vi "Update DI DAQ IO Group.vi"(7 "dCVT DAQDict":T2, 8 "error in (no error)":errorcluster, 9 "DI in":bool[](array[boolean]), 10 "DI channels":T3[](array[typedef]), 11 "DIO ClusterArray":T1[](array[typedef])) -> (0 "error out":errorcluster, 3 "DIO ClusterArray out":T1[](array[typedef]), 5 "dCVT DAQDict out":T2)   [LabVIEW 2020, in "DAQDict.lvlib"]
uses:
  DAQDict.lvlib
  support/IONameNode--cluster.ctl
  <vilib>/TELLC/Dynamic CVT API/TD Dynamic CVT DVR--ref.ctl
  support/DIO ClusterArray Element--cluster.ctl
  support/BRS_DI - New.ctl
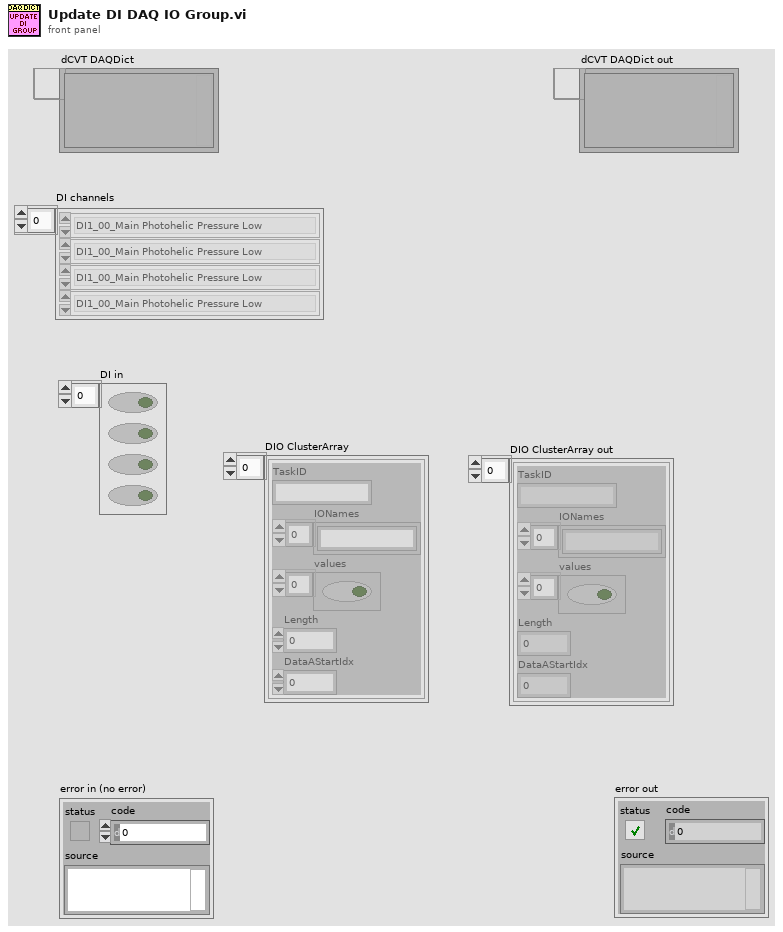
[diagram p1: front panel]
types:
  T1 = typedef "DIO ClusterArray Element--cluster.ctl" = cluster{"TaskID":string, "IONames":string[], "values":bool[], "Length":i32, "DataAStartIdx":i32}
  T2 = typedef "TD Dynamic CVT DVR--ref.ctl" = refnum<data-value>
  T3 = typedef "BRS_DI - New.ctl" = enum16{"DI1_00_Main Photohelic Pressure Low", "DI1_01_Main Photohelic Pressure High", "DI1_02_Main E-Stop Circuit OK", "DI1_03_EMO Circuit OK", "DI1_04_Nitrogen Top Valve Open", "DI1_05_Nitrogen Bottom Valve Open", "DI1_06_Nitrogen Pressure OK", "DI1_07_CDA Pressure OK", "DI1_08_Vacuum OK", "DI1_09_Aligner Home", "DI1_10_Aligner Reticle Present", "DI1_11_Main Door Interlock Solenoid Closed", "DI1_12_Main Door Closed", "DI1_13_Main Robot $ALARM_STOP", "DI1_14_Main Robot $IN_HOME", "DI1_15_Main Robot $PERI_RDY", "DI1_16_Main Robot $TCP_OPEN", "DI1_17_Main End Eff Open", "DI1_18_Main End Eff Closed", "DI1_19_Main Reticle Presence sensor-Arm-Right", "DI1_20_Spare_1", "DI1_21_Main Reticle Presence sensor-Arm-Left", "DI1_22_EXP1 XFR Reticle Present", "DI1_23_EXP2 XFR Reticle Present", "DI1_24_Main Robot $EXT (External Mode ON)", "DI1_25_Main Robot $PRO_ACT (Program Active)", "DI1_26_Main Robot $PRO_MOVE (Motion Active)", "DI1_27_Main Robot Spare1", "DI1_28_Main Robot Spare2", "DI1_29_Main Robot Spare3", "DI1_30_Spare_2", "DI1_31_Spare_3", "DI2_00_ASML_RSP LP 1 Pod Presence", "DI2_01_Spare_4", "DI2_02_ASML_RSP LP 2 Pod Presence", "DI2_03_Spare_5", "DI2_04_ASML_RSP LP 3 Pod Presence", "DI2_05_Spare_6", "DI2_06_Spare_7", "DI2_07_Manual Loadport 1 Pod Present", "DI2_08_Manual Loadport 1 Pod Capture", "DI2_09_Manual Loadport 1 Arm in Open Position", "DI2_10_Manual Loadport 1 Arm in Closed Position", "DI2_11_Manual Loadport 1 Lid Capture", "DI2_12_Manual Loadport 1 Door Closed", "DI2_13_Manual Loadport 1 Reticle Present", "DI2_14_Manual Loadport 1 Lid Present on Arm", "DI2_15_MLP Spare Input", "DI2_16_Pod Buffer Inbound Pod Present", "DI2_17_Pod Buffer Outbound Pod Present", "DI2_18_Pod Buffer Door Closed", "DI2_19_Pod Buffer Light Curtain OK", "DI2_20_Pod Buffer Light Curtain Misc Input", "DI2_21_Pod Buffer Gripper Pod Present", "DI2_22_Pod Buffer Gripper open", "DI2_23_Pod Buffer Gripper closed", "DI2_24_FFU Pressure sensor 1", "DI2_25_FFU Pressure sensor 2", "DI2_26_FFU Pressure sensor 3", "DI2_27_FFU Pressure sensor 4", "DI2_28_FFU Pressure sensor 5", "DI2_29_FFU Pressure sensor 6", "DI2_30_FFU Pressure sensor 7", "DI2_31_FFU Pressure sensor 8", "DI3_00_Exp1 Photohelic Pressure Low", "DI3_01_Exp1 Photohelic Pressure High", "DI3_02_Main E-Stop Circuit OK", "DI3_03_Spare_1", "DI3_04_Exp1 Door Interlock Solenoid Closed", "DI3_05_Exp1 Door Closed", "DI3_06_Spare_2", "DI3_07_Spare_3", "DI3_08_Spare_4", "DI3_09_Spare_5", "DI3_10_Exp1 End Eff Open", "DI3_11_Exp1 End Eff Closed", "DI3_12_Exp1 Reticle Presence sensor-Arm-Right", "DI3_13_Exp1 Robot $ALARM_STOP", "DI3_14_Exp1 Robot $IN_HOME", "DI3_15_Exp1 Robot $PERI_RDY", "DI3_16_Exp1 Robot $TCP_OPEN", "DI3_17_Exp1 Reticle Presence sensor-Arm-Left", "DI3_18_Exp1 FFU Pressure sensor 1", "DI3_19_Exp1 FFU Pressure sensor 2", "DI3_20_Exp1 FFU Pressure sensor 3", "DI3_21_Exp1 FFU Pressure sensor 4", "DI3_22_Exp1 FFU Pressure sensor 5", "DI3_23_Exp1 FFU Pressure sensor 6", "DI3_24_Exp1 Robot $EXT (External Mode ON)", "DI3_25_Exp1 Robot $PRO_ACT (Program Active)", "DI3_26_Exp1 Robot $PRO_MOVE (Motion Active)", "DI3_27_Exp1 FFU Pressure sensor 7", "DI3_28_Exp1 FFU Pressure sensor 8", "DI3_29_Exp1 output Spare 1", "DI3_30_Exp1 output Spare 2", "DI3_31_Exp1 output Spare 3"}
  T4 = typedef "IONameNode--cluster.ctl" = cluster{"IOName":string, "value":bool, "IO Type":enum16{"N/A", "DI", "DO"}, "TaskID":string, "data Idx":i32}
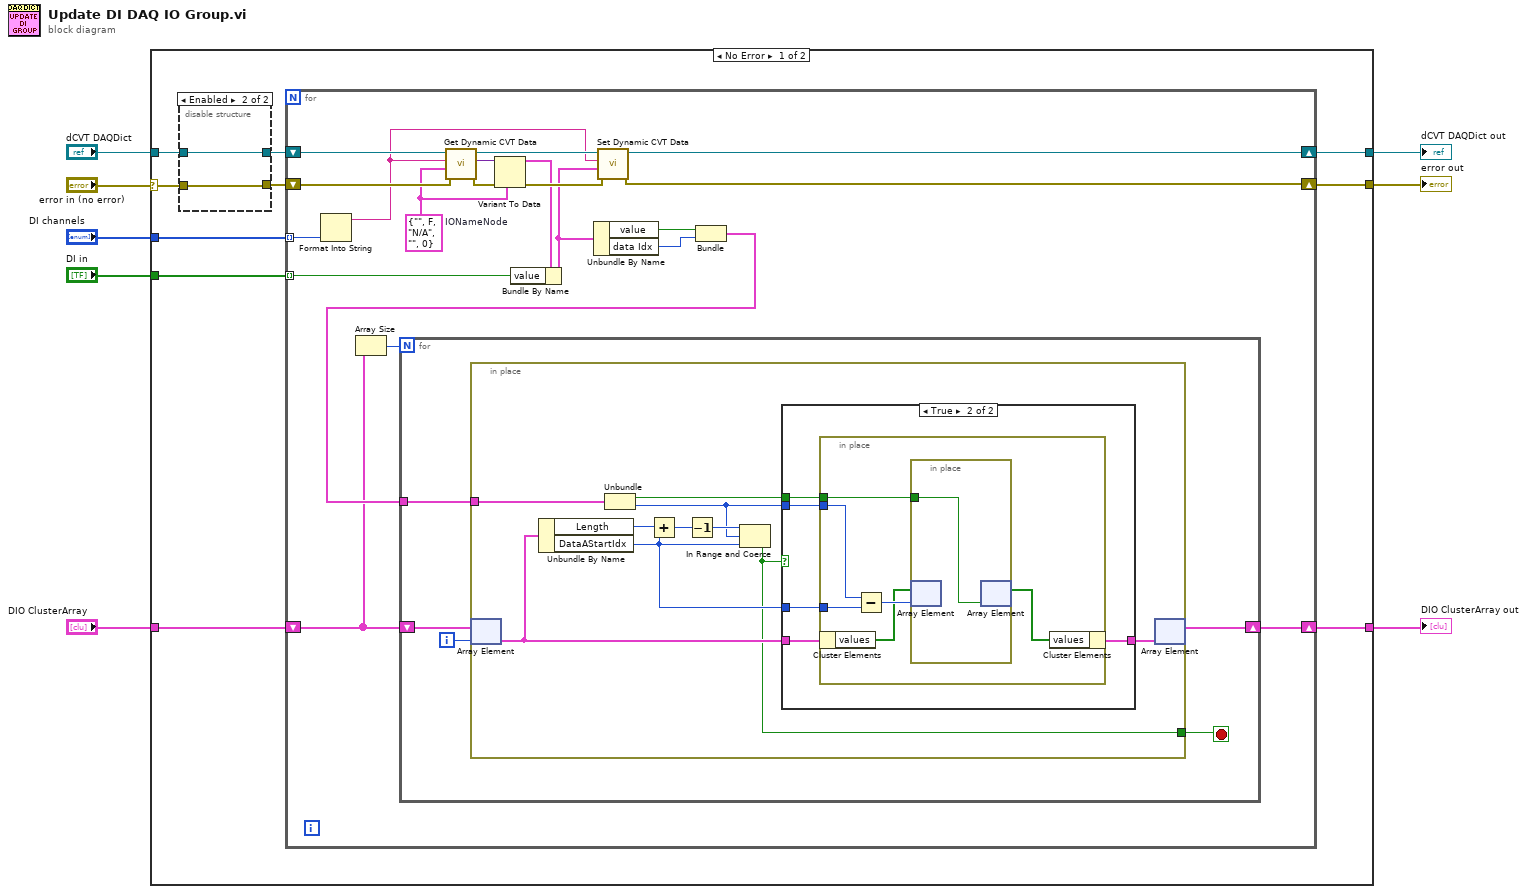
[diagram p0: block diagram]
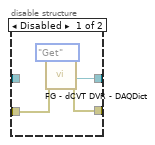
[diagram p2: hidden frame]
diagram:
  n1 = case shown="No Error" "error in (no error)" {
    selector: "error in (no error)" -> [w17 w75]
    tunnel: [w15 w75] -> w8
    tunnel: "DI channels" -> [w16 _]
    tunnel: [w14 w74] -> w5
    tunnel: "dCVT DAQDict" -> [w12 w74]
    tunnel: "DI in" -> [w11 _]
    tunnel: "DIO ClusterArray" -> [w10 w73]
    tunnel: [w9 w73] -> w1
    frame No Error {
      n2 = disable-structure shown="Enabled" {
        disable-tunnel: [w21 w23] -> w18
        disable-tunnel: w17 -> [w20 w23]
        disable-tunnel: [w19 w24] -> w13
        disable-tunnel: w12 -> [_ w24]
        frame Disabled {
          n3 = call "FG - dCVT DVR - DAQDict.vi"("error in (no error)"=w20, "Action (Get)"=enum16{"Init", "Get", "Set"}."Get") -> ("dCVT DAQDict out"=w19:T2, "error out"=w21:errorcluster)  [unwired: 7 in]
        }
        frame Enabled {
        }
      }
      n4 = for {
        shift-right: [w36] -> w14
        shift-left: w13 -> [w44]
        shift-right: [w34] -> w15
        shift-left: w18 -> [w43]
        tunnel: w16 -> [w42] mode=indexing
        tunnel: w11 -> [w30] mode=indexing
        shift-right: [w25] -> w9
        shift-left: w10 -> [w27]
        w39 = T4 {"IOName"="", "value"=FALSE, "IO Type"=enum."N/A", "TaskID"="", "data Idx"=0}  # IONameNode
        n5 = Format Into String(w42) -> (resulting string=w32:string)  [unwired: 3 in, 1 out]
        n6 = Array Size(array=w27) -> (size(s)=w26:i32)
        n7 = call <vilib>:"Get Dynamic CVT Data.vi"("error in (no error)"=w43, "default value (empty variant)"=w39, "DataName"=w32, "dCVT DVR"=w44) -> ("error out"=w40:errorcluster, "value"=w41:variant, "dCVT DVR out"=w37:T2)  [unwired: 4 in, 1 out]
        n8 = Variant To Data(error in=w40, type=w39, Variant=w41) -> (data=w33:T4, error out=w35:errorcluster)
        n9 = Bundle By Name(cluster=w33, "value"=w30) -> (w31:T4)
        n10 = Unbundle By Name(w31) -> ("value"=w38:bool, "data Idx"=w29:i32)
        n11 = call <vilib>:"Set Dynamic CVT Data.vi"("error in (no error)"=w35, "value"=w31, "DataName"=w32, "dCVT DVR"=w37) -> ("error out"=w34:errorcluster, "dCVT DVR out"=w36:T2)  [unwired: 5 in, 1 out]
        n12 = Bundle("value"=w38, "data Idx"=w29) -> (w28:cluster{"value":bool, "data Idx":i32})  [unwired: 1 in]
        n13 = for {
          N: w26 -> [_]
          tunnel: w28 -> [w49]
          shift-right: [w47] -> w25
          shift-left: w27 -> [w48]
          i -> [w46]
          stop <- w45 stop-if-true
          n14 = in-place {
            in-place-border: w49 -> [w56]
            in-place-border: [w51] -> w45
            n15 = in-place-array #1(w48, w46) -> (w52:T1)
            n16 = Unbundle By Name(w52) -> ("Length"=w58:i32, "DataAStartIdx"=w53:i32)
            n17 = Unbundle(w56) -> ("value"=w55:bool, "data Idx"=w54:i32)
            n18 = Add(x=w58, y=w53) -> (x+y=w59:i32)
            n19 = Decrement(x=w59) -> (x-1=w57:i32)
            n20 = In Range and Coerce(upper limit=w57, x=w54, lower limit=w53) -> (In Range?=w51:bool)  [unwired: 1 out]
            n21 = case shown="True" w51 {
              tunnel: w55 -> [_ w64]
              tunnel: w54 -> [_ w63]
              tunnel: w52 -> [w60 w65]
              tunnel: w53 -> [_ w62]
              tunnel: [w60 w61] -> w50
              frame False {
              }
              frame True {
                n22 = in-place {
                  in-place-border: w64 -> [w67]
                  in-place-border: w63 -> [w69]
                  in-place-border: w62 -> [w70]
                  n23 = in-place-cluster #2(w65) -> ("values"=w68:bool[])
                  n24 = Subtract(x=w69, y=w70) -> (x-y=w71:i32)
                  n25 = in-place {
                    in-place-border: w67 -> [w72]
                    n26 = in-place-array #3(w68, w71) -> ()  [unwired: 1 out]
                    n27 = in-place-array #3(w72) -> (w66:bool[])  [unwired: 1 out]
                  }
                  n28 = in-place-cluster #2("values"=w66) -> (w61:T1)
                }
              }
            }
            n29 = in-place-array #1(w50) -> (w47:T1[])  [unwired: 1 out]
          }
        }
      }
    }
    frame Error {
    }
  }
  "error out" <- w8
  "dCVT DAQDict out" <- w5
  "DIO ClusterArray out" <- w1
